vi "430_TCP_compound query test_v1.vi"() -> ()   [LabVIEW 2011]
panel:
  out "refnum out":refnum<file>
  out "file check":errorcluster
  in  "file path (use dialog)":path
  in  "save":bool
  out "status":i32
  in  "Timeout":i32=1000
  out "field":string
  out "Query check":errorcluster
  out "Response":string
  in  "Command":string
  out "Init Response":string
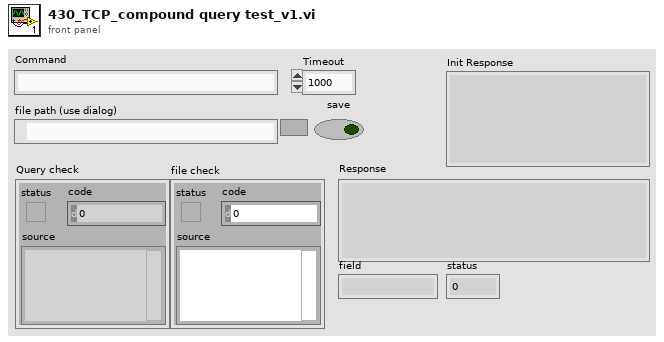
[diagram p1: front panel]
types:
  T1 = enum16{"open", "replace", "create", "open or create", "replace or create", "replace or create with confirmation"}
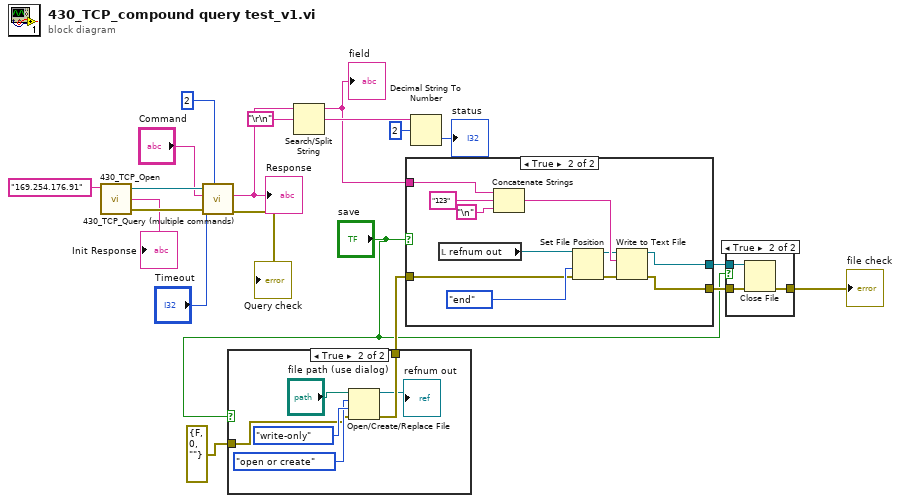
[diagram p0: block diagram]
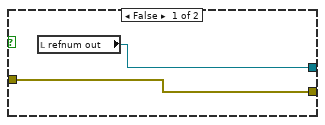
[diagram p4: hidden frame]
diagram:
  n1 = call "430_TCP_Open.vi"("IP Address"="169.254.176.91") -> ("connection ID"=w18:refnum<k5>, "Init Response"=→"Init Response":string, "error out"=w19:errorcluster)  [unwired: 5 in]
  n2 = call "430_TCP_Query (multiple commands).vi"("Number of\nquerys"=2 ("Number of\nquerys"), "error in (no error)"=w19, "Timeout"="Timeout", "Command"="Command", "connection ID"=w18) -> ("error out"=→"Query check":errorcluster, "Response"=w14:string)  [unwired: 2 in, 3 out]
  "Response" <- w14
  n3 = case shown="True" "save" {
    tunnel: [w21 w24] -> w11
    tunnel: errorcluster {"status"=FALSE, "code"=0, "source"=""} ("error out") -> [w21 w22]
    frame False {
    }
    frame True {
      n4 = Open/Create/Replace File(file path (use dialog)="file path (use dialog)", error in=w22, operation (0:open)=T1."open or create", access (0:read/write)=enum16{"read/write", "read-only", "write-only"}."write-only") -> (refnum out=→"refnum out":refnum<file>, error out=w24:errorcluster)  [unwired: 2 in, 1 out]
    }
  }
  n5 = Search/Split String(string=w14, search string/char (-)="\r\n") -> (substring before match=w1:string, match + rest of string=w3:string)  [unwired: 1 in, 1 out]
  "field" <- w1
  n6 = case shown="True" "save" {
    tunnel: [w29 w35] -> w9
    tunnel: w11 -> [w29 w36]
    tunnel: [w28 w34] -> w8
    tunnel: w1 -> [_ w30]
    frame False {
      n7 = local read "refnum out"() -> (w28:refnum<file>)
    }
    frame True {
      n8 = local read "refnum out"() -> (w33:refnum<file>)
      n9 = Concatenate Strings(w30, "123" ("string"), "\n") -> (w40:string)
      n10 = Set File Position(refnum=w33, from (0:start)=enum16{"start", "end", "current"}."end", error in=w36) -> (refnum out=w39:refnum<file>, error out=w37:errorcluster)  [unwired: 1 in]
      n11 = Write to Text File(file (use dialog)=w39, text=w40, error in=w37) -> (refnum out=w34:refnum<file>, error out=w35:errorcluster)  [unwired: 1 in, 1 out]
    }
  }
  n12 = Decimal String To Number(string=w3, offset=2) -> (number=→"status":i32)  [unwired: 1 in, 1 out]
  n13 = case shown="True" "save" {
    tunnel: [w41 w44] -> w10
    tunnel: w9 -> [w41 w43]
    tunnel: w8 -> [_ w42]
    frame False {
    }
    frame True {
      n14 = Close File(refnum=w42, error in=w43) -> (error out=w44:errorcluster)  [unwired: 1 out]
    }
  }
  "file check" <- w10
